vi "CalculateTrajectory.vi"(8 "error in (no error)":errorcluster, 11 "MatrixOfPoints":T1) -> (0 "error out":errorcluster, 1 "z":dbl[](array[numeric]), 2 "y":dbl[](array[numeric]), 3 "x":dbl[](array[numeric]))   [LabVIEW 2014, in "Manipulator.lvclass"]
uses:
  Manipulator.lvclass
  <vilib>/Analysis/Matrix/Datatypes/RealMatrix.ctl
  <vilib>/Analysis/Matrix/NI_Matrix.lvlib
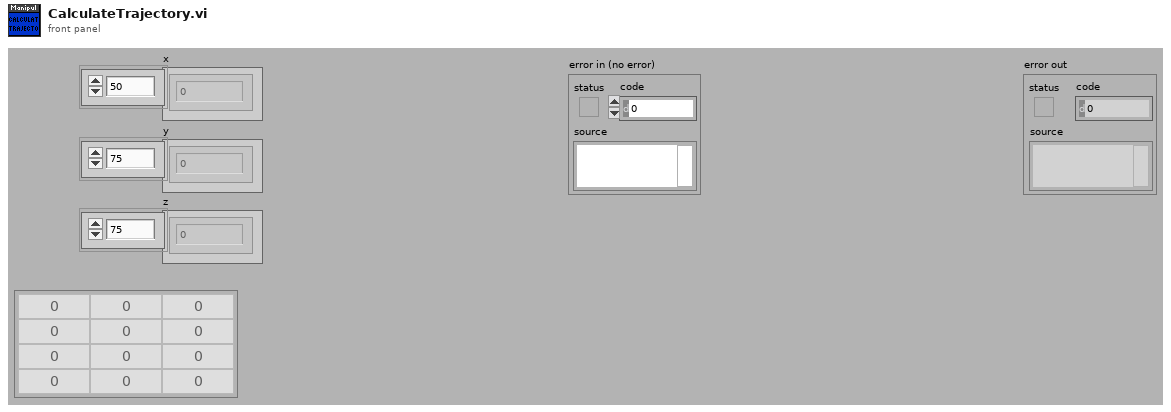
[diagram p1: front panel]
types:
  T1 = typedef "NI_Matrix.lvlib/RealMatrix.ctl" = dbl[][]
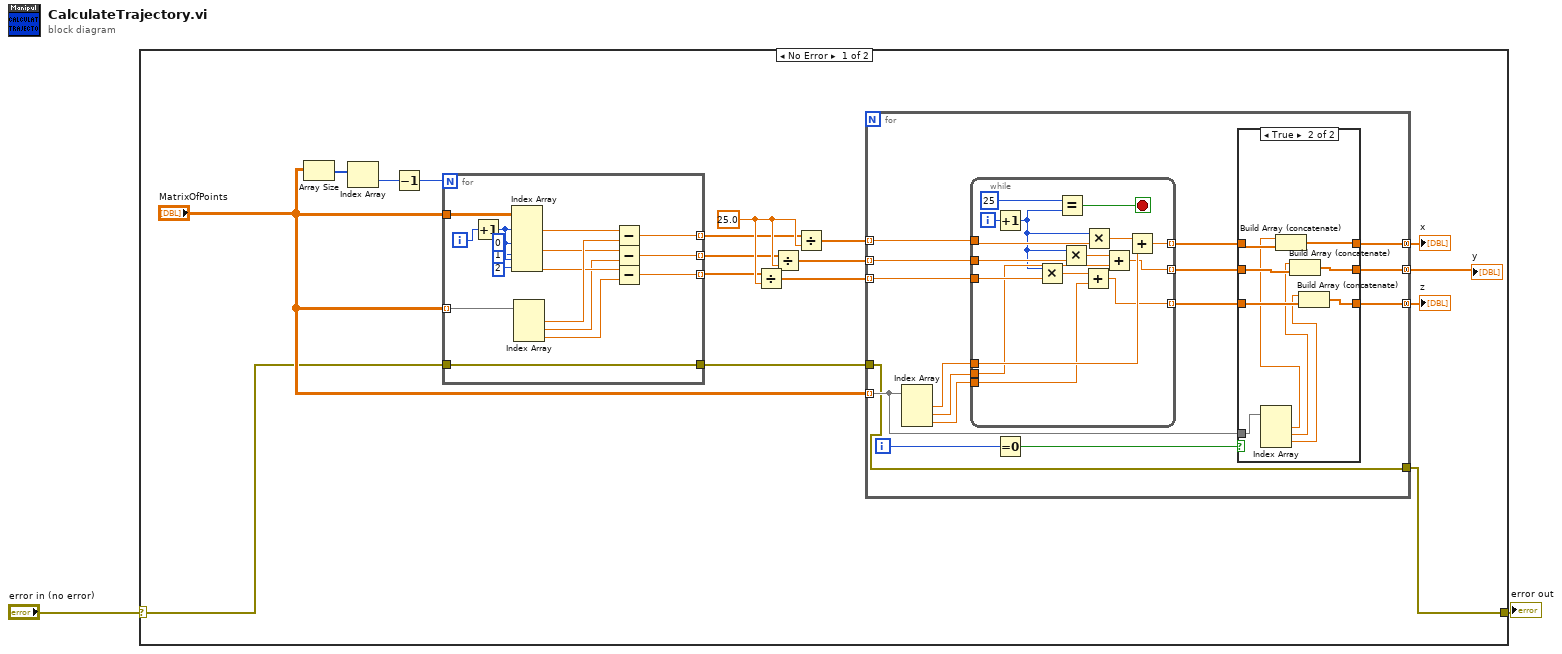
[diagram p0: block diagram]
diagram:
  n1 = case shown="No Error" "error in (no error)" {
    selector: "error in (no error)" -> [w5 w82]
    tunnel: [w3 w82] -> w1
    frame No Error {
      w17 = 25.0
      n2 = Array Size(array="MatrixOfPoints") -> (size(s)=w19:i32[])
      n3 = Index Array(array=w19) -> (element=w18:i32)  [unwired: 1 in]
      n4 = Decrement(x=w18) -> (x-1=w13:i32)
      n5 = for {
        N: w13 -> [_]
        tunnel: "MatrixOfPoints" -> [w81]
        tunnel: "MatrixOfPoints" -> [w78] mode=indexing
        tunnel: [w73] -> w16 mode=indexing
        tunnel: [w67] -> w15 mode=indexing
        tunnel: [w66] -> w14 mode=indexing
        tunnel: [w65] -> w4
        tunnel: w5 -> [w65]
        i -> [w80]
        n6 = Increment(x=w80) -> (x+1=w79:i32)
        n7 = Index Array(array=w81, index (row) #1=w79, index (col) #1=0 ("disabled index (col)"), index (row) #2=w79, index (col) #2=1 ("disabled index (col)"), index (row) #3=w79, index (col) #3=2 ("disabled index (col)")) -> (element #1=w77:dbl, element #2=w71:dbl, element #3=w70:dbl)
        n8 = Index Array(array=w78) -> (element #1=w72:dbl, element #2=w69:dbl, element #3=w68:dbl)  [unwired: 3 in]
        n9 = Subtract(x=w77, y=w72) -> (x-y=w73:dbl)
        n10 = Subtract(x=w71, y=w69) -> (x-y=w67:dbl)
        n11 = Subtract(x=w70, y=w68) -> (x-y=w66:dbl)
      }
      n12 = Divide(x=w14, y=w17) -> (x/y=w9:dbl[])
      n13 = Divide(x=w15, y=w17) -> (x/y=w10:dbl[])
      n14 = Divide(x=w16, y=w17) -> (x/y=w11:dbl[])
      n15 = for {
        tunnel: "MatrixOfPoints" -> [w21] mode=indexing
        tunnel: w11 -> [w32] mode=indexing
        tunnel: w10 -> [w31] mode=indexing
        tunnel: w9 -> [w30] mode=indexing
        tunnel: [w25] -> w8 mode=concatenating
        tunnel: [w24] -> w7 mode=concatenating
        tunnel: [w23] -> w6 mode=concatenating
        tunnel: w4 -> [w20]
        tunnel: [w20] -> w3
        i -> [w29]
        n16 = Index Array(array=w21) -> (element #1=w35:dbl, element #2=w34:dbl, element #3=w33:dbl)  [unwired: 3 in]
        n17 = while {
          tunnel: w35 -> [w57]
          tunnel: w34 -> [w54]
          tunnel: w33 -> [w53]
          tunnel: w32 -> [w62]
          tunnel: w31 -> [w61]
          tunnel: w30 -> [w59]
          tunnel: [w52] -> w28 mode=indexing
          tunnel: [w51] -> w27 mode=indexing
          tunnel: [w50] -> w26 mode=indexing
          i -> [w60]
          stop <- w64 stop-if-true
          n18 = Increment(x=w60) -> (x+1=w49:i32)
          n19 = Multiply(x=w49, y=w59) -> (x*y=w55:dbl)
          n20 = Equal?(x=25 ("y"), y=w49) -> (x = y?=w64:bool)
          n21 = Multiply(x=w49, y=w61) -> (x*y=w56:dbl)
          n22 = Add(x=w55, y=w53) -> (x+y=w50:dbl)
          n23 = Multiply(x=w49, y=w62) -> (x*y=w58:dbl)
          n24 = Add(x=w56, y=w54) -> (x+y=w51:dbl)
          n25 = Add(x=w58, y=w57) -> (x+y=w52:dbl)
        }
        n26 = Equal To 0?(x=w29) -> (x = 0?=w22:bool)
        n27 = case shown="True" w22 {
          tunnel: w28 -> [w38 w47]
          tunnel: w27 -> [w37 w44]
          tunnel: w26 -> [w36 w42]
          tunnel: [w38 w46] -> w25
          tunnel: [w37 w45] -> w24
          tunnel: [w36 w43] -> w23
          tunnel: w21 -> [_ w48]
          frame False {
          }
          frame True {
            n28 = Index Array(array=w48) -> (element #1=w41:dbl, element #2=w40:dbl, element #3=w39:dbl)  [unwired: 3 in]
            n29 = Build Array (concatenate)(w41, w47) -> (w46:dbl[])
            n30 = Build Array (concatenate)(w40, w44) -> (w45:dbl[])
            n31 = Build Array (concatenate)(w39, w42) -> (w43:dbl[])
          }
        }
      }
      "x" <- w8
      "y" <- w7
      "z" <- w6
    }
    frame Error {
    }
  }
  "error out" <- w1
